vi "Acquisition Done.vi"(8 "error in (no error)":errorcluster, 11 "Simulated Camera in":refnum<class "Simulated Camera.lvclass">) -> (0 "error out":errorcluster, 2 "Acquisition Done":bool, 3 "Simulated Camera out":refnum<class "Simulated Camera.lvclass">)   [LabVIEW 2019, in "Simulated Camera.lvclass"]
uses:
  Simulated Camera.lvclass
  Simulated Camera.lvclass/Simulated Camera.ctl
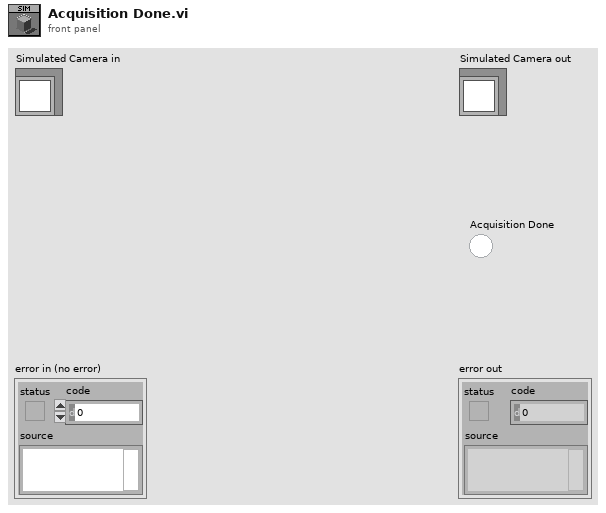
[diagram p1: front panel]
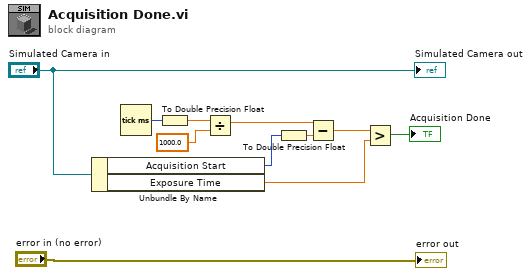
[diagram p0: block diagram]
diagram:
  n1 = Unbundle By Name("Simulated Camera in") -> ("Acquisition Start"=w9:i32, "Exposure Time"=w7:dbl)
  n2 = Tick Count (ms)() -> (millisecond timer value=w6:u32)
  n3 = To Double Precision Float(number=w6) -> (double precision float=w4:dbl)
  n4 = Divide(x=w4, y=1000.0 ("x")) -> (x/y=w10:dbl)
  n5 = To Double Precision Float(number=w9) -> (double precision float=w8:dbl)
  n6 = Subtract(x=w10, y=w8) -> (x-y=w3:dbl)
  n7 = Greater?(x=w3, y=w7) -> (0:→"Acquisition Done":bool)
  "error out" <- "error in (no error)"
  "Simulated Camera out" <- "Simulated Camera in"
